vi "Real FFT(half complex).vi"(0 "X":dbl[](array[numeric]) format="%0.2f") -> (1 "FFT {X}":dbl[](array[numeric]) format="%0.2f", 2 "error":i32)   [LabVIEW 2010, in "NI_AALPro.lvlib"]
doc: "Computes the Real Fast Fourier Transform (FFT) or the Real Discrete Fourier Transform (DFT) of the input sequence <B>X</B>."
uses:
  NI_AALPro.lvlib
  lvanlys.dll
panel:
  # "Real (half complex) FFT"
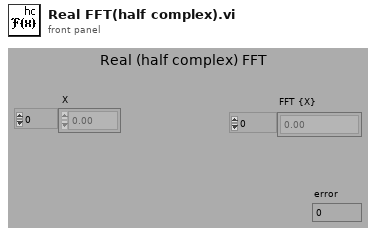
[diagram p1: front panel]
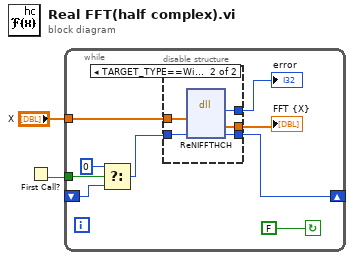
[diagram p0: block diagram]
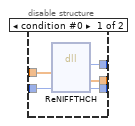
[diagram p2: hidden frame]
diagram:
  n1 = First Call?() -> (First Call?: T/F=w1:bool)
  n2 = while {
    shift-left: _ -> [w6]
    shift-right: [w4] -> _
    tunnel: "X" -> [w11]
    tunnel: w1 -> [w7]
    stop <- FALSE continue-if-true
    n3 = Select(t=0, s=w7, f=w6) -> (s? t:f=w5:i64)
    n4 = disable-structure shown="TARGET_TYPE==Windows||TARGET_TYPE==Mac||TARGET_TYPE==Unix" {
      disable-tunnel: w11 -> [w16 w21]
      disable-tunnel: [w15 w20] -> w10
      disable-tunnel: [w14 w19] -> w9
      disable-tunnel: w5 -> [w13 w18]
      disable-tunnel: [w12 w17] -> w4
      frame condition #0 {
        n5 = dll-call lib="C:/Program Files/National Instruments/LabVIEW 2010/resource/lvanlys.dll" fn="ReNIFFTHCH"("xH"=w16, w13) -> ("return type"=w15:i32, "yH"=w14:dbl[], w12:i32)  [unwired: 5 in, 2 out]
      }
      frame condition #1 (active) {
        n6 = dll-call lib="C:/Program Files/National Instruments/LabVIEW 2010/resource/lvanlys.dll" fn="ReNIFFTHCH"("xH"=w21, "arg3"=w18) -> ("return type"=w20:i32, "yH"=w19:dbl[], "arg3"=w17:i64)  [unwired: 5 in, 2 out]
      }
    }
    "FFT {X}" <- w9
    "error" <- w10
  }
